vi "Send.vi"(8 "error in (no error)":errorcluster, 11 "Plugin Generic Command in":refnum<class "Plugin Handler Command.lvclass">) -> (0 "error out":errorcluster, 3 "Plugin Generic Command out":refnum<class "Plugin Handler Command.lvclass">)   [LabVIEW 2011, in "Plugin Handler Command.lvclass"]
uses:
  Plugin Handler Command.lvclass
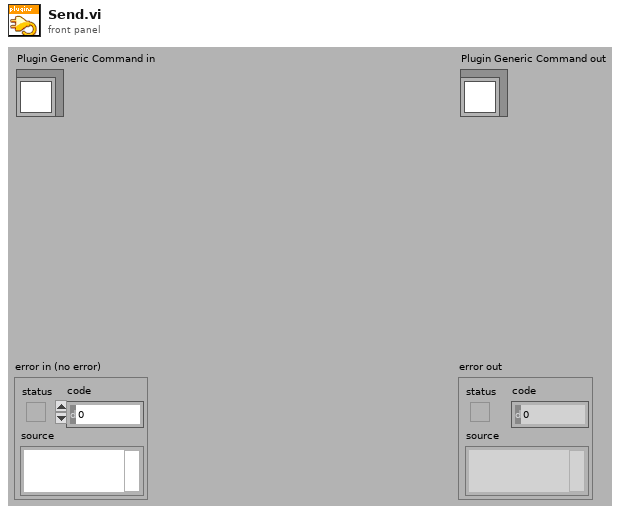
[diagram p1: front panel]
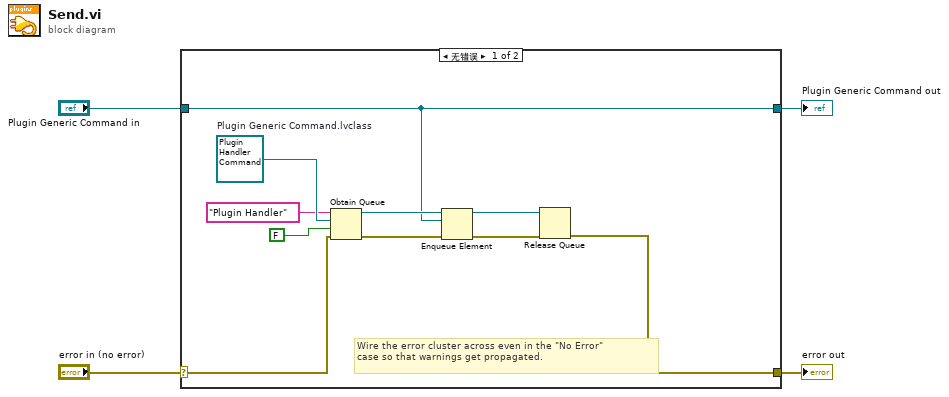
[diagram p0: block diagram]
diagram:
  n1 = case shown="无错误" "error in (no error)" {
    selector: "error in (no error)" -> [w6 w16]
    tunnel: [w5 w16] -> w3
    tunnel: [w9 w15] -> w1
    tunnel: "Plugin Generic Command in" -> [w9 w15]
    frame No Error {
      w14 = refnum<class "Plugin Handler Command.lvclass"> refnum  # Plugin Generic Command.lvclass
      # "Wire the error cluster across even in the \"No Error\"\ncase so that warnings get propagated."
      n2 = Obtain Queue(name (unnamed)="Plugin Handler", element data type=w14, create if not found? (T)=FALSE, error in (no error)=w6) -> (queue out=w11:refnum<queue>, error out=w10:errorcluster)  [unwired: 1 in, 1 out]
      n3 = Enqueue Element(queue=w11, element=w9, error in (no error)=w10) -> (queue out=w8:refnum<queue>, error out=w7:errorcluster)  [unwired: 1 in, 1 out]
      n4 = Release Queue(queue=w8, error in (no error)=w7) -> (error out=w5:errorcluster)  [unwired: 1 in, 2 out]
    }
    frame Error {
    }
  }
  "error out" <- w3
  "Plugin Generic Command out" <- w1
